vi "QCP_SetDbl.vi"(6 "Add if New?":bool, 8 "error in":errorcluster, 9 "Value":dbl, 10 "Name":string, 11 "QCP_DevRef_In":T1) -> (0 "error out":errorcluster, 3 "QCP_DevRef_Out":T1)   [LabVIEW 2016]
uses:
  <userlib>/836-libraries/System/QCP_V2/QCPSupportCode/QCP_RefNum.ctl
  <userlib>/836-libraries/System/QCP_V2/QCPSupportCode/QCPData.ctl
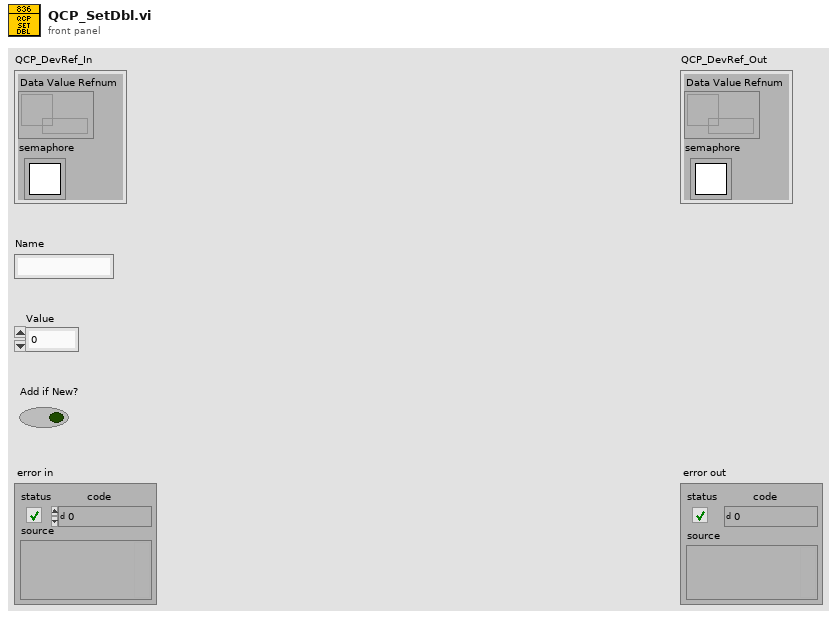
[diagram p1: front panel]
types:
  T1 = typedef "QCP_RefNum.ctl" = cluster{"Data Value Refnum":refnum<data-value>, "semaphore":T2}
  T2 = typedef "Semaphore RefNum" = refnum<k1>
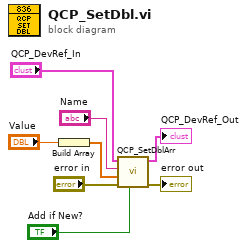
[diagram p0: block diagram]
diagram:
  n1 = Build Array("Value") -> (w1:dbl[])
  n2 = call <userlib>:"QCP_SetDblArr.vi"("Add if New?"="Add if New?", "error in"="error in", "Values"=w1, "Name"="Name", "QCP_DevRef_In"="QCP_DevRef_In") -> ("error out"=→"error out":errorcluster, "QCP_DevRef_Out"=→"QCP_DevRef_Out":T1)  [unwired: 5 in]
